vi "AddTextToJPEGfile.vi"(5 "[user-specified font]":T3, 6 "quality (80)":i32=80, 7 "desired font(Application)":T2(ring)=enum."System Font", 8 "error in (no error)":errorcluster, 9 "textOrigin":cluster{"x":i16, "y":i16}, 10 "text":string, 11 "pathIn":path) -> (0 "error out":errorcluster)   [LabVIEW 2015]
uses:
  <vilib>/picture/picture.llb/imagedata.ctl
panel:
  out "image data":T1
  out "2D Picture":picture
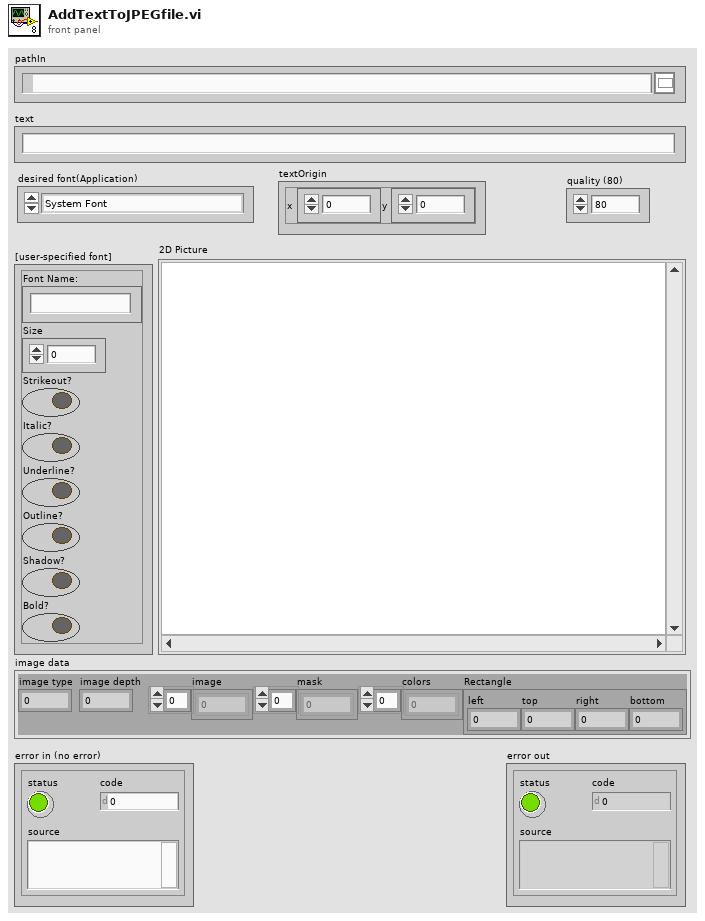
[diagram p1: front panel]
types:
  T1 = typedef "imagedata.ctl" = cluster{"image type":i32, "image depth":i32, "image":u8[], "mask":u8[], "colors":u32[], "Rectangle":cluster{"left":i16, "top":i16, "right":i16, "bottom":i16}}
  T2 = enum16{"User-specified Font", "Application Font", "System Font", "Dialog Font"}
  T3 = cluster{"Font Name:":string, "Size":i16, "Strikeout?":bool, "Italic?":bool, "Underline?":bool, "Outline?":bool, "Shadow?":bool, "Bold?":bool}
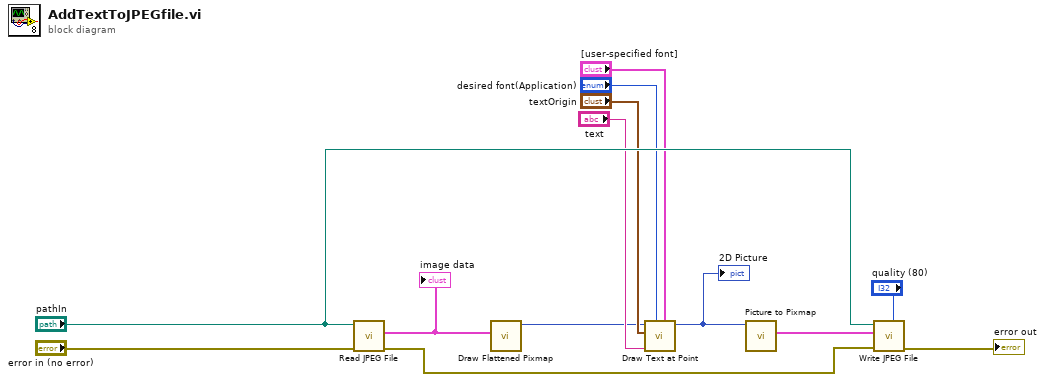
[diagram p0: block diagram]
diagram:
  n1 = call <vilib>:"Read JPEG File.vi"("error in (no error)"="error in (no error)", "path to JPEG file"="pathIn") -> ("error out"=w11:errorcluster, "image data"=w1:T1)  [unwired: 7 in, 1 out]
  "image data" <- w1
  n2 = call <vilib>:"Draw Flattened Pixmap.vi"("image data"=w1) -> ("new picture"=w2:picture)  [unwired: 8 in]
  n3 = call <vilib>:"Draw Text at Point.vi"("[user-specified font]"="[user-specified font]", "desired font(Application)"="desired font(Application)", "text"="text", "origin"="textOrigin", "picture"=w2) -> ("new picture"=w7:picture)  [unwired: 5 in, 1 out]
  "2D Picture" <- w7
  n4 = call <vilib>:"Picture to Pixmap.vi"("picture"=w7) -> ("image data"=w8:T1)  [unwired: 9 in, 1 out]
  n5 = call <vilib>:"Write JPEG File.vi"("quality (80)"="quality (80)", "error in (no error)"=w11, "image data"=w8, "path to JPEG file"="pathIn") -> ("error out"=→"error out":errorcluster)  [unwired: 6 in, 1 out]
